vi "03 Vaporizador.vi"() -> ()   [LabVIEW 2021]
panel:
  in  "Masa":u64
  in  "Sustancia":dbl(ring)=2261.11 items=["Agua"=2261.11, "Alcohol Etílico"=854.34, "Benceno"=394.87]
  out "Gauge":dbl(knob) scale=0.0..20000.0
  in  "Detener":bool
  # "VAPORIZADOR"
  # "CONDICIONES"
  # "kJ"
  # "Desarrollado por:\n     Semillero Electroquimica e Innovación Ambiental - SEIA"
  # "g"
  # "Calor Necesario"
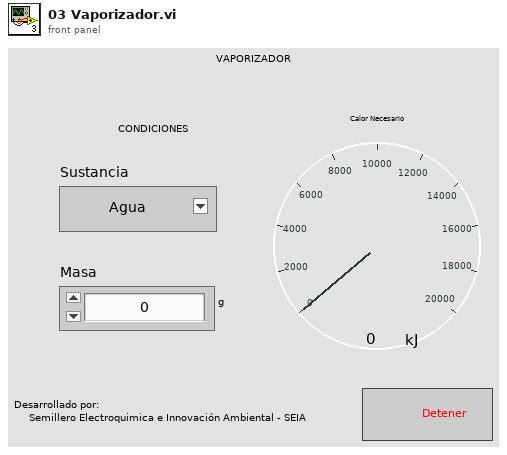
[diagram p1: front panel]
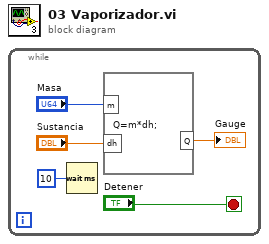
[diagram p0: block diagram]
diagram:
  n1 = while {
    stop <- "Detener" stop-if-true
    n2 = Wait (ms)(milliseconds to wait=u32 10) -> ()  [unwired: 1 out]
    n3 = formula code="Q=m*dh;"("dh"="Sustancia", "m"="Masa") -> ("Q"=→"Gauge":dbl)
  }
